vi "sW&col situation.vi"(0 "Overal CURV(mm)":dbl format="%#_2g", 1 "SW array in":dbl[](array[numeric]), 2 "curv and Sw setting":T1, 3 "col count":i8, 4 "capture":bool=TRUE, 5 "error in (no error)":errorcluster) -> (14 "curv sit":bool, 15 "right SideWall":bool, 16 "Left SideWall":bool, 18 "Elapsed Time (s)":dbl, 19 "error out":errorcluster)   [LabVIEW 2019]
uses:
  <vilib>/measure/mamon.llb/Trigger Detection for 1 Channel.vi
  <vilib>/measure/NI_MAPro.lvlib
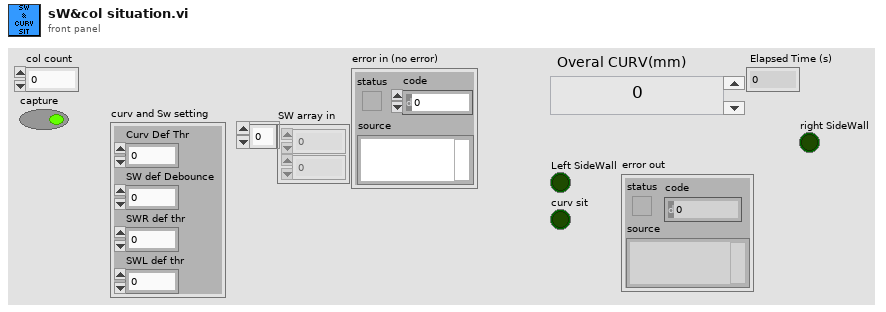
[diagram p1: front panel]
types:
  T1 = cluster{"Curv Def Thr":dbl, "SW def Debounce":dbl, "SWR def thr":dbl, "SWL def thr ":dbl}
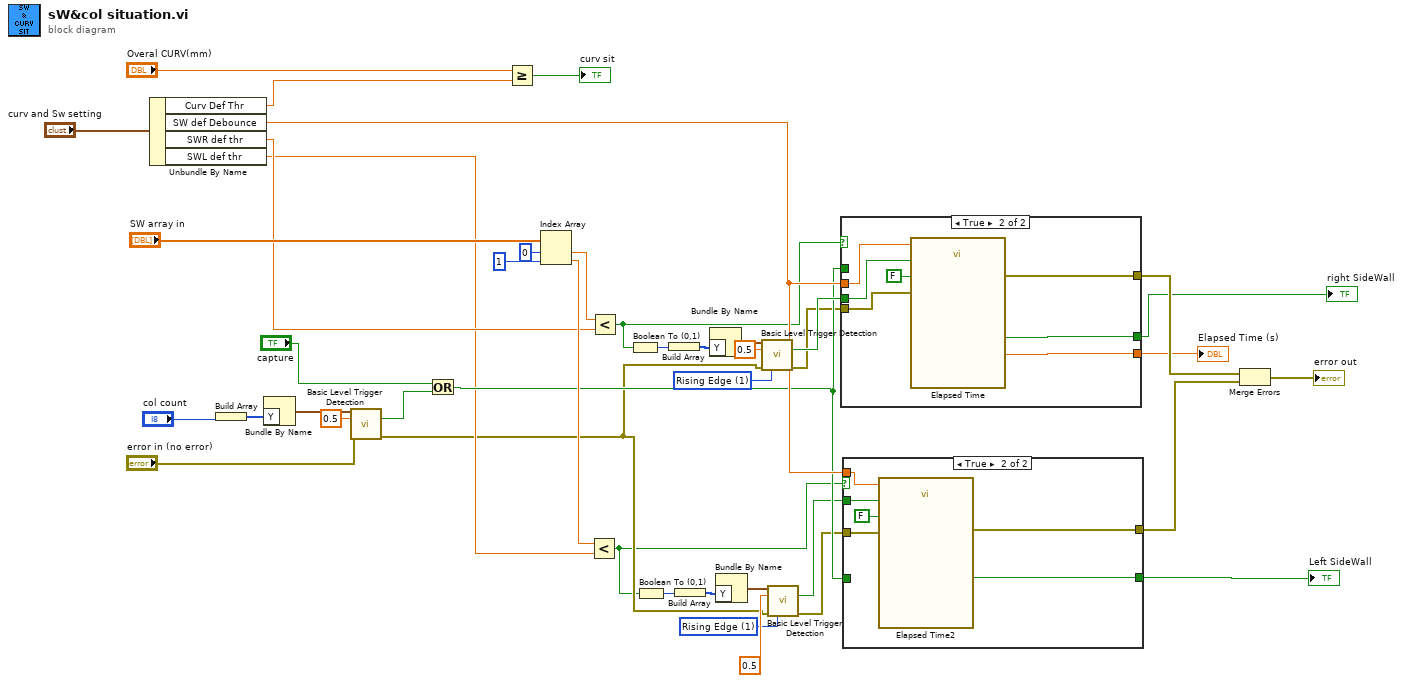
[diagram p0: block diagram]
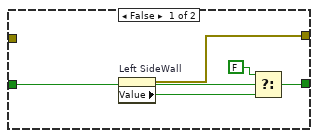
[diagram p2: hidden frame]
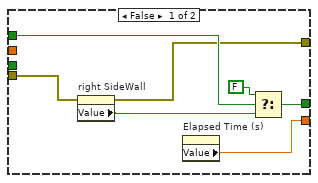
[diagram p3: hidden frame]
diagram:
  w5 = u16 1 items=["Falling Edge", "Rising Edge"] ("trigger slope")
  w38 = u16 1 items=["Falling Edge", "Rising Edge"] ("trigger slope")
  n1 = Unbundle By Name("curv and Sw setting") -> ("Curv Def Thr"=w30:dbl, "SW def Debounce"=w29:dbl, "SWR def thr"=w15:dbl, "SWL def thr"=w10:dbl)
  n2 = Build Array("col count") -> (w27:i8[])
  n3 = Bundle By Name("Y"=w27) -> (w26:waveform(i8))  [unwired: 1 in]
  n4 = call-poly <vilib>:"Basic Level Trigger Detection.vi"("signal in"=w26, "level"=0.5, "error in (no error)"="error in (no error)") -> ("trigger detected?"=w23:bool, "error out"=w4:errorcluster)  [unwired: 10 in, 1 out]
  n5 = Or(x="capture", y=w23) -> (x .or. y?=w22:bool)
  n6 = Greater Or Equal?(x="Overal CURV(mm)", y=w30) -> (x >= y?=→"curv sit":bool)
  n7 = Index Array(array="SW array in", index #1=0 ("index"), index #2=1 ("index")) -> (element #1=w37:dbl, element #2=w35:dbl)
  n8 = Less?(x=w35, y=w10) -> (x < y?=w3:bool)
  n9 = Less?(x=w37, y=w15) -> (x < y?=w13:bool)
  n10 = Boolean To (0,1)(Boolean=w13) -> (0, 1=w14:i16)
  n11 = Boolean To (0,1)(Boolean=w3) -> (0, 1=w8:i16)
  n12 = Build Array(w14) -> (w40:i16[])
  n13 = Build Array(w8) -> (w6:i16[])
  n14 = Bundle By Name("Y"=w40) -> (w39:waveform(i16))  [unwired: 1 in]
  n15 = Bundle By Name("Y"=w6) -> (w7:waveform(i16))  [unwired: 1 in]
  n16 = call-poly <vilib>:"Basic Level Trigger Detection.vi"("signal in"=w39, "level"=0.5, "error in (no error)"=w4, "trigger slope"=w38) -> ("trigger detected?"=w36:bool, "error out"=w20:errorcluster)  [unwired: 9 in, 1 out]
  n17 = call-poly <vilib>:"Basic Level Trigger Detection.vi"("signal in"=w7, "level"=0.5, "error in (no error)"=w4, "trigger slope"=w5) -> ("trigger detected?"=w2:bool, "error out"=w1:errorcluster)  [unwired: 9 in, 1 out]
  n18 = case shown="True" w13 {
    tunnel: w36 -> [_ w57]
    tunnel: w29 -> [_ w56]
    tunnel: [w49 w55] -> w12
    tunnel: w22 -> [w48 _]
    tunnel: w20 -> [w45 w54]
    tunnel: [w44 w53] -> w19
    tunnel: [w47 w52] -> w16
    frame False {
      n19 = property on="right SideWall" class="Bool (strict)"(error in=w45) -> (error out=w44:errorcluster, "Value"=w46:bool)  [unwired: 1 in, 1 out]
      n20 = property on="Elapsed Time (s)" class="DigNum (strict)"() -> ("Value"=w47:dbl)  [unwired: 2 in, 2 out]
      n21 = Select(t=FALSE, s=w48, f=w46) -> (s? t:f=w49:bool)
    }
    frame True {
      n22 = call "Elapsed Time"("Time Target (s)"=w56, "Reset"=w57, "Auto Reset"=FALSE, "error in (no error)"=w54) -> ("Elapsed Time (s)"=w52:dbl, "Time has Elapsed"=w55:bool, "error out"=w53:errorcluster)  [unwired: 8 in, 5 out]
    }
  }
  "Elapsed Time (s)" <- w16
  "right SideWall" <- w12
  n23 = case shown="True" w3 {
    tunnel: [w61 w68] -> w34
    tunnel: w29 -> [_ w67]
    tunnel: w22 -> [w59 _]
    tunnel: [w58 w66] -> w18
    tunnel: w2 -> [_ w65]
    tunnel: w1 -> [_ w63]
    frame False {
      n24 = property on="Left SideWall" class="Bool (strict)"() -> (error out=w58:errorcluster, "Value"=w60:bool)  [unwired: 2 in, 1 out]
      n25 = Select(t=FALSE, s=w59, f=w60) -> (s? t:f=w61:bool)
    }
    frame True {
      n26 = call "Elapsed Time2"("Time Target (s)"=w67, "Reset"=w65, "Auto Reset"=FALSE, "error in (no error)"=w63) -> ("Time has Elapsed"=w68:bool, "error out"=w66:errorcluster)  [unwired: 8 in, 6 out]
    }
  }
  "Left SideWall" <- w34
  n27 = Merge Errors(w19, w18) -> (→"error out":errorcluster)
